vi "Destroy Tree Branch.vi"(10 "error in":errorcluster, 11 "Tree in":refnum<class "Tree.lvclass">) -> (2 "error out":errorcluster, 3 "Root":variant)   [LabVIEW 2019, in "Tree.lvclass"]
uses:
  Tree.lvclass
  Tree.lvclass/Tree.ctl
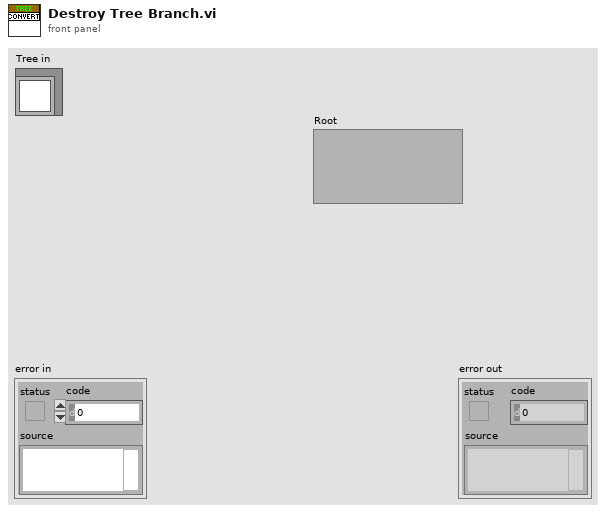
[diagram p1: front panel]
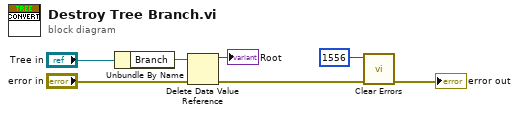
[diagram p0: block diagram]
diagram:
  n1 = Unbundle By Name("Tree in") -> ("Branch"=w6:refnum<data-value>)
  n2 = Delete Data Value Reference(data value reference=w6, error in="error in") -> (data value=→"Root":variant, error out=w3:errorcluster)
  n3 = call <vilib>:"Clear Errors.vi"("error in (no error)"=w3, "specific error code to clear (0: all)"=1556) -> ("error out"=→"error out":errorcluster)  [unwired: 4 in, 1 out]
